vi "Validate Range.vi"(8 "error in (no error)":errorcluster, 10 "Range":T1, 11 "Varian Continuous in":refnum<class "Varian Continuous.lvclass">) -> (0 "error out":errorcluster, 2 "Validated Range":T1, 3 "Varian Continuous out":refnum<class "Varian Continuous.lvclass">)   [LabVIEW 2009, in "Varian Continuous.lvclass"]
doc: "Coerce the range to be within this Scanner's physical limits."
uses:
  Varian Continuous.lvclass
  Scanner/Range.ctl
  Scanner/Scanner.lvclass
  Instruments/Varian Magnet/Varian Max Field.vi
  Instruments/Varian Magnet/Varian Magnet.lvclass
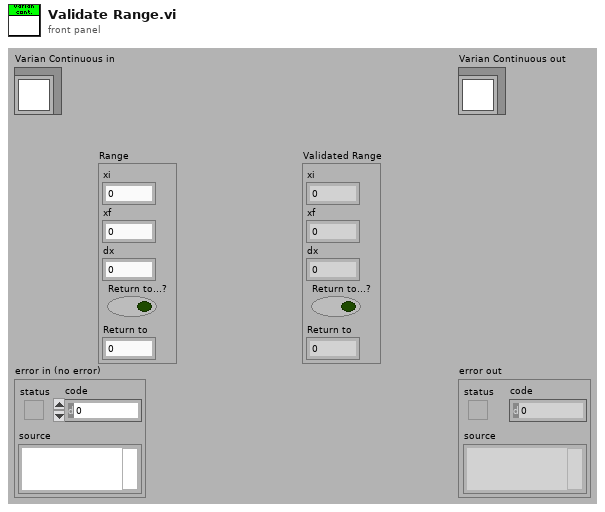
[diagram p1: front panel]
types:
  T1 = typedef "Scanner.lvclass/Range.ctl" = cluster{"xi":dbl, "xf":dbl, "dx":dbl, "Return to...?":bool, "Return to":dbl}
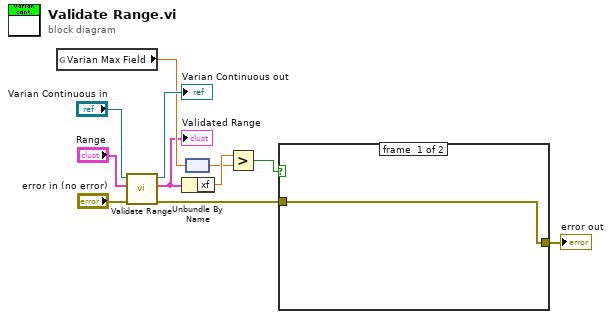
[diagram p0: block diagram]
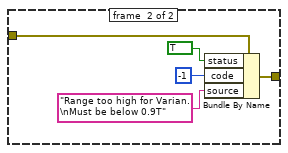
[diagram p2: hidden frame]
diagram:
  n1 = global read "Varian Max Field.vi" "Varian Max Field"() -> (w6:dbl[unit])
  n2 = call-parent "Validate Range.vi"("error in (no error)"="error in (no error)", "Range"="Range", "Scanner in"="Varian Continuous in") -> ("error out"=w3:errorcluster, "Validated Range"=w2:T1, "Scanner out"=→"Varian Continuous out":refnum<class "Varian Continuous.lvclass">)  [unwired: 6 in]
  "Validated Range" <- w2
  n3 = Unbundle By Name(w2) -> ("xf"=w7:dbl)
  n4 = node(w6) -> (w5:dbl)
  n5 = Greater?(x=w7, y=w5) -> (0:w4:bool)
  n6 = case shown="True" w4 {
    tunnel: w3 -> [w12 w17]
    tunnel: [w12 w13] -> w1
    frame #0 {
    }
    frame #1 {
      n7 = Bundle By Name(cluster=w17, "status"=TRUE, "code"=-1, "source"="Range too high for Varian.\nMust be below 0.9T") -> (w13:errorcluster)
    }
  }
  "error out" <- w1
